vi "FailureDescription.vi"(8 "error in (no error)":errorcluster, 10 "Actual":variant, 11 "IsRefnum in":refnum<class "IsRefnum.lvclass">) -> (0 "error out":errorcluster, 2 "Failure Description":string, 3 "IsRefnum out":refnum<class "IsRefnum.lvclass">)   [LabVIEW 2019, in "Constraint.lvlib" / "IsRefnum.lvclass"]
doc: "Return the second part of the scentence \"Failed asserting that ...\""
uses:
  IsRefnum.lvclass
  <vilib>/Utility/Data Type/NI_Data Type.lvlib
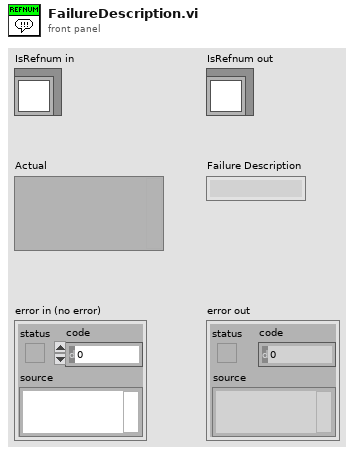
[diagram p1: front panel]
types:
  T1 = typedef "NI_Data Type.lvlib/Refnum Type.ctl" = enum16{"NotARefnum", "UnknownRefnum", "Generic", "Datalog", "ByteStream", "Device", "Occurence", "TCPNetConnection", "Auto", "Menu", "Imaq", "Hardware", "DataSocket", "Visa", "IVI", "UDPNetConnection", "Notifier", "Queue", "Irda", "EventReg", "DotNet", "UserEvent", "Callback", "UNUSED_EMPTY_POSITION", "BlueToothNetConnection", "LVObjApp", "LVObjVI", "LVObjUnknown", "GenericClass", "UserDefinedRefnumTag", "DataValue", "RT FIFO", "TDMS File", "PythonSessionRefnum"}
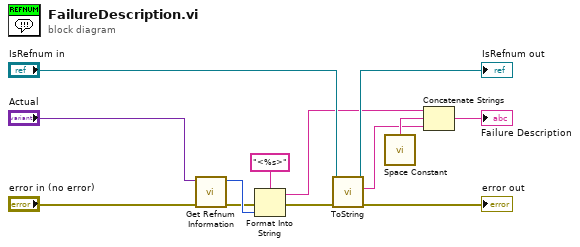
[diagram p0: block diagram]
diagram:
  n1 = call <vilib>:"Get Refnum Information.vi"("error in (no error)"="error in (no error)", "variant"="Actual") -> ("error out"=w2:errorcluster, "reference type"=w4:T1)  [unwired: 6 in, 2 out]
  n2 = Format Into String(format string="<%s>", error in=w2, w4) -> (resulting string=w5:string, error out=w1:errorcluster)  [unwired: 1 in]
  n3 = call-dynamic "ToString.vi"("error in (no error)"=w1, "IsRefnum in"="IsRefnum in") -> ("error out"=→"error out":errorcluster, "String"=w12:string, "IsRefnum out"=→"IsRefnum out":refnum<class "IsRefnum.lvclass">)  [unwired: 7 in]
  n4 = call <vilib>:"Space Constant.vi"() -> ("String"=w13:string)
  n5 = Concatenate Strings(w5, w13, w12) -> (→"Failure Description":string)
